vi "Get Attributes.vi"(8 "error in (no error)":errorcluster, 9 "tag index":i32, 11 "xml structure in":T1) -> (0 "error out":errorcluster, 1 "Attributes":cluster{"Keys":string[], "Values":string[]}, 3 "xml structure out":T1)   [LabVIEW 2011]
uses:
  XML Structure - Cluster.ctl
  XML Tag Type - Enum.ctl
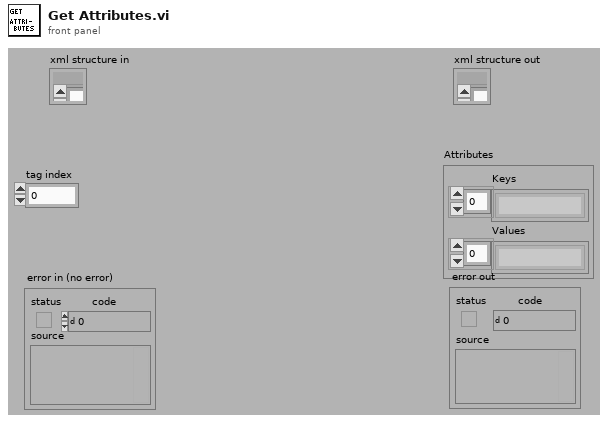
[diagram p1: front panel]
types:
  T1 = typedef "XML Structure - Cluster.ctl" = cluster{"tags":string[], "tag names":string[], "tag type":T2[], "offset":i32[], "close tag index":i32[], "xml":string, "Children":cluster{"children":i32[]}[], "parent index":i32[]}
  T2 = typedef "XML Tag Type - Enum.ctl" = enum16{"start tag", "empty tag", "end tag"}
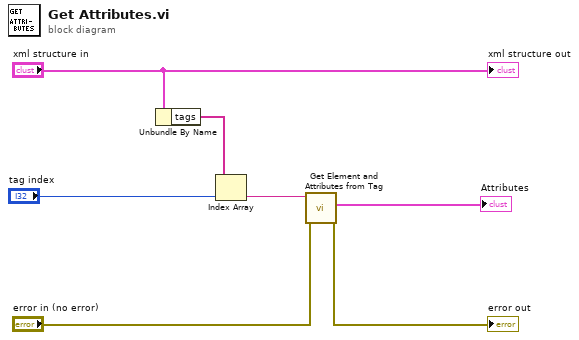
[diagram p0: block diagram]
diagram:
  n1 = Unbundle By Name("xml structure in") -> ("tags"=w5:string[])
  n2 = Index Array(array=w5, index="tag index") -> (element=w4:string)
  n3 = call "Get Element and Attributes from Tag.vi"("error in (no error)"="error in (no error)", "tag with attributes"=w4) -> ("error out"=→"error out":errorcluster, "Attributes"=→"Attributes":cluster{"Keys":string[], "Values":string[]})  [unwired: 6 in, 2 out]
  "xml structure out" <- "xml structure in"
